vi "SubjectFactory.vi"(11 "Enum":enum16{"Subject 1", "Subject 2"}(ring)) -> (3 "Normal Proxy.lvlib:Subject.lvclass":refnum<class "Subject.lvclass">)   [LabVIEW 2014, in "Normal Proxy.lvlib"]
uses:
  Normal Proxy.lvlib
  Subject/Subject.lvclass
  RealSubject1/RealSubject1.lvclass
  RealSubject2/RealSubject2.lvclass
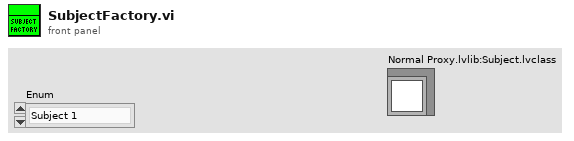
[diagram p1: front panel]
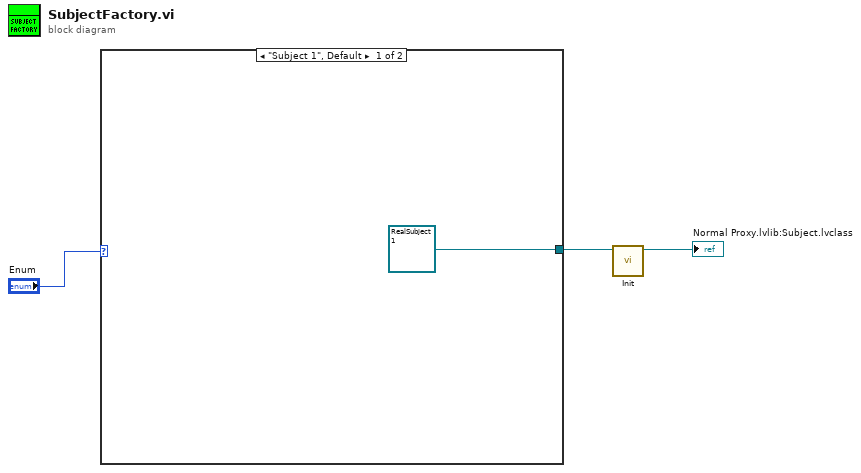
[diagram p0: block diagram]
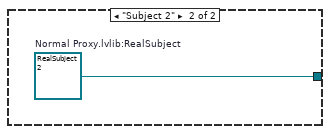
[diagram p2: hidden frame]
diagram:
  n1 = case shown="\"Subject 1\", Default" "Enum" {
    tunnel: [refnum<class "RealSubject1.lvclass"> refnum ("Normal Proxy.lvlib:RealSubject1") w5] -> w2
    frame "Subject 1", Default {
    }
    frame "Subject 2" {
      w5 = refnum<class "RealSubject2.lvclass"> refnum  # Normal Proxy.lvlib:RealSubject
    }
  }
  n2 = call-dynamic "Init.vi"("Subject in"=w2) -> ("Subject out"=→"Normal Proxy.lvlib:Subject.lvclass":refnum<class "Subject.lvclass">)  [unwired: 9 in, 1 out]
